vi "Dispersion measurements.vi"() -> ()   [LabVIEW 2015]
uses:
  <vilib>/express/express arith-compare/Formula/XNode/ExpressFormulaBlockNode.xnode
  <instrlib>/Rohde&Schwarz Vector Network Analyzer/Rohde&Schwarz Vector Network Analyzer.lvlib
panel:
  in  "Minimum field (Oe)":dbl min=-1000.0 max=1000.0
  in  "Maximum field (Oe)":dbl=1.0 min=0.0 max=1000.0
  out "Amplifier LinMag gain":dbl
  in  "Power amplifier LinMag gain (if 0, it will be calculated)":dbl min=0.0 max=20.0
  in  "Stop frequency (Hz)":dbl=15000000000.0 min=0.0 max=20000000000.0
  in  "Start frequency (Hz)":dbl=100000.0 min=0.0 max=20000000000.0
  in  "1 Hz < IFBW < 1MHz (10 kHz default)":dbl=10000.0 min=1.0 max=10000000.0
  in  "-20 dB < Power < 20 dB (0 dB default)":dbl min=-20.0 max=20.0
  in  "Delay time along ther sample (ps)":dbl min=0.0 max=1000.0
  out "DMM reading":dbl=5.649249
  out "Current field point":i32=98
  in  "DMM's connection":refnum<visa-resource-name>="Multimeter"
  in  "Choose the folder where the field dependencies of S-parameters and Z will be saved":path=path "C:/Users/ZJUcomposite/Desktop/Tests"
  in  "HMF's connection":refnum<visa-resource-name>="Generator"
  in  "VNA's connection":refnum<visa-resource-name>="ZNB-VNA"
  in  "Coil resistance > 0 (Ohm)":dbl=8.38 min=0.1 max=1000.0
  in  "Coil inductance > 0 (H)":dbl=0.32 min=0.0 max=100.0
  in  "Number of field points":i32=2 min=2 max=1000 step=1
  in  "Volltage to field coefficient > 0 (Oe/V)":dbl=4.29 min=0.0 max=1000.0
  in  "Max input voltage for the amplifier (0<V<2)":dbl=1.5 min=0.0 max=10.0
  in  "Number of frequency points":i32=5000 min=3 max=20000
  in  "VNA's port(s) used for measurements":string(combo)="S21"
  # "The procedure measures the frequency dispersions of S-parameters and Z for the specified magnetic fields.\n\nVNA must be already calibrated before the measurements. The procedure will not change the calibration but you can   modify IFBW and power. The frequency measurement range must be within the calibration range. \n\nThe measured fields must be within the maximum (+/-) field range.\n\nThe voltage to field coefficient (Oe/V) must be found from the coil calibration.\n\nThe delay time along the sample must be found separately.\n\nThe coil resistance R and inductance L must be larger than zero. Measure them by a digital multimeter (DMM).\n\nPlease check the maximum input voltage max V allowed for your waveform amplifier. Also the ratio maxV / R must be below the current rate of your waveform amplifier.  \n\n******************************************\nDmitriy Makhnovskiy@Hangzhou December 2018\nSensing Materials Technology Ltd, UK\nE-mail: contact@sensmattech.co.uk"
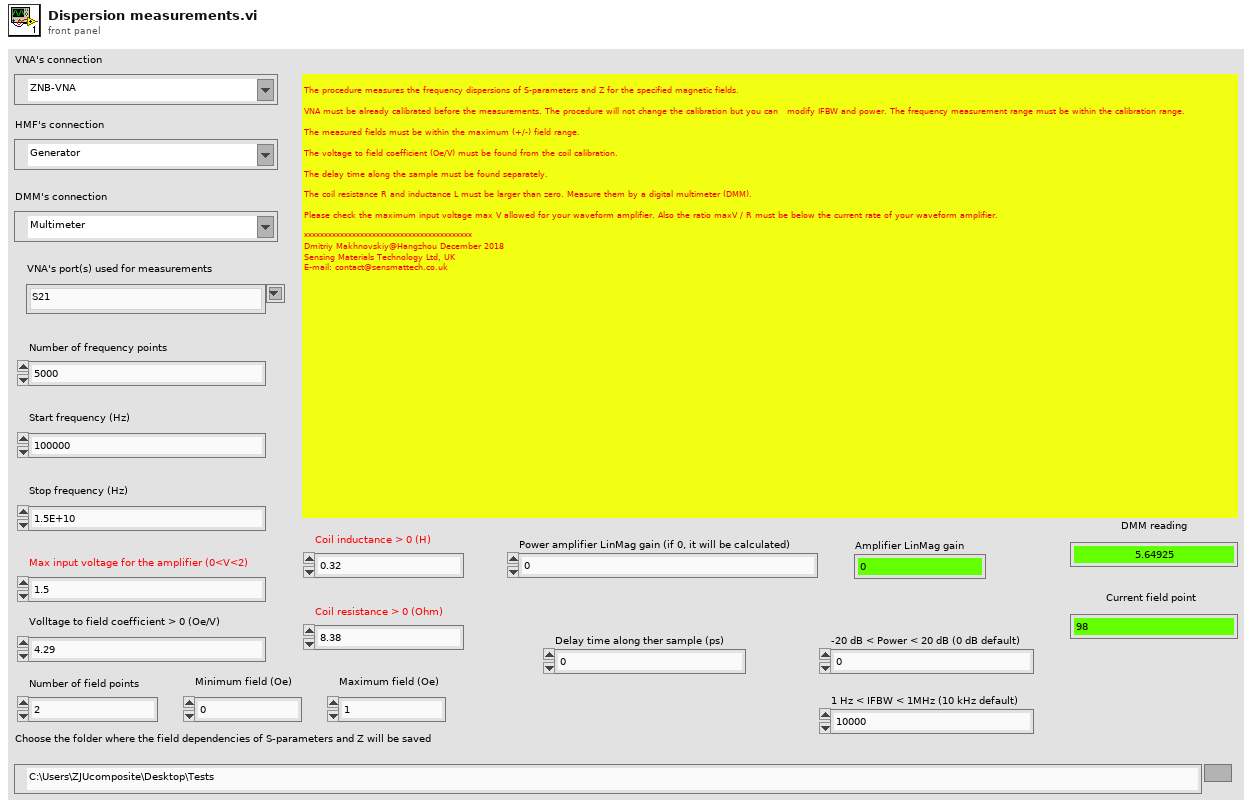
[diagram p1: front panel]
types:
  T1 = typedef "NI_Matrix.lvlib/RealMatrix.ctl" = dbl[][]
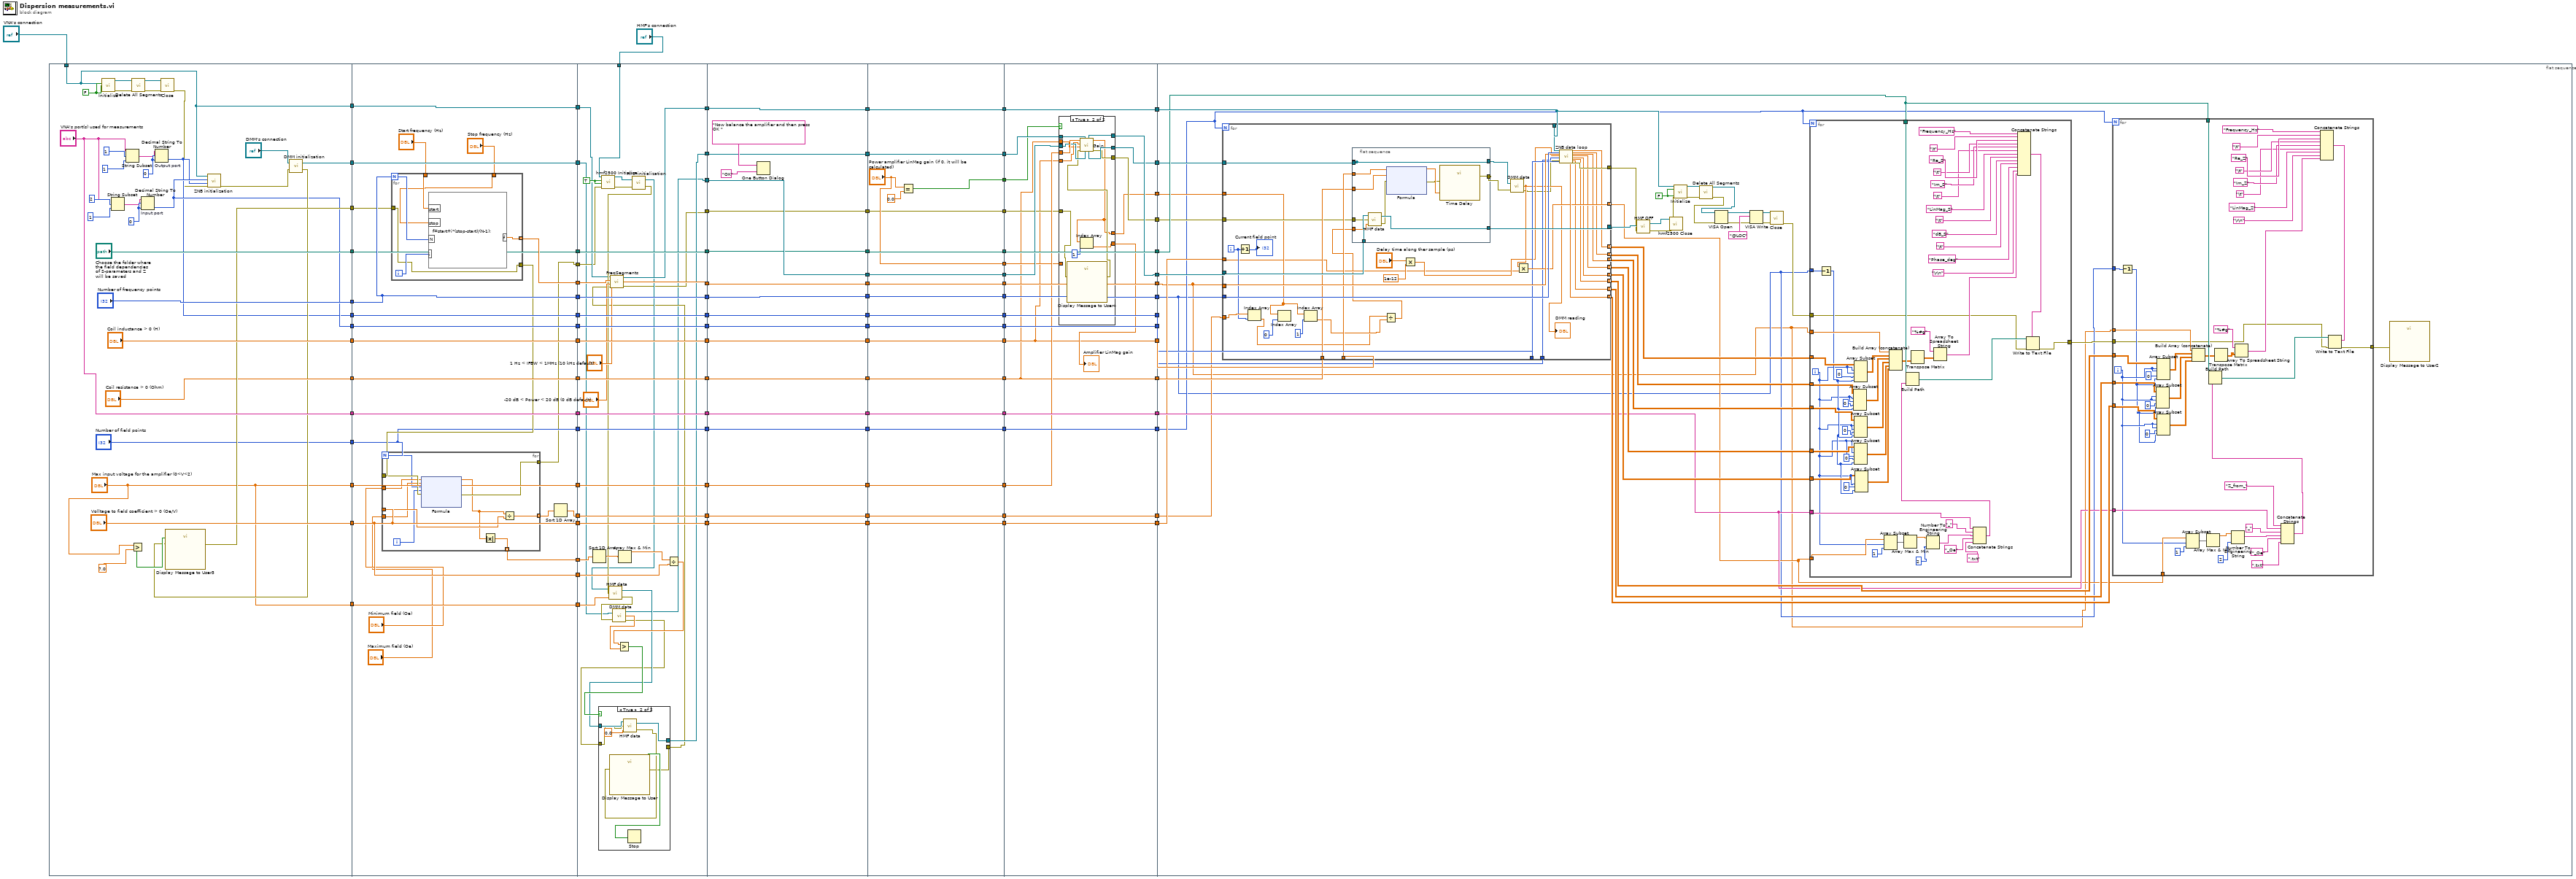
[diagram p0: block diagram]
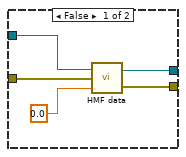
[diagram p2: hidden frame]
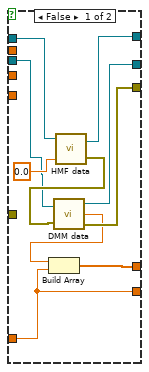
[diagram p3: hidden frame]
diagram:
  n1 = flat-sequence {
    tunnel: [w108] -> w92
    tunnel: ["VNA's port(s) used for measurements"] -> w89
    tunnel: "VNA's connection" -> [w108]
    tunnel: ["Number of frequency points"] -> w87
    tunnel: ["Coil inductance > 0 (H)"] -> w84
    tunnel: ["Coil resistance > 0 (Ohm)"] -> w81
    tunnel: ["Max input voltage for the amplifier (0<V<2)"] -> w78
    tunnel: ["Volltage to field coefficient > 0 (Oe/V)"] -> w75
    tunnel: ["Choose the folder where the field dependencies of S-parameters and Z will be saved"] -> w72
    tunnel: [w118] -> w71
    tunnel: [w113] -> w68
    tunnel: [w111] -> w65
    tunnel: [w110] -> w62
    tunnel: ["Number of field points"] -> w61
    tunnel: ["Max input voltage for the amplifier (0<V<2)"] -> w53
    tunnel: [w156] -> w100
    tunnel: [w153] -> w98
    tunnel: [w135] -> w96
    tunnel: [w155] -> w93
    tunnel: w92 -> [w155]
    tunnel: [w154] -> w90
    tunnel: w89 -> [w154]
    tunnel: w87 -> [w153]
    tunnel: [w152] -> w85
    tunnel: w84 -> [w152]
    tunnel: [w151] -> w82
    tunnel: w81 -> [w151]
    tunnel: [w139] -> w79
    tunnel: w78 -> [w139]
    tunnel: [w137] -> w76
    tunnel: w75 -> [w137]
    tunnel: [w150] -> w73
    tunnel: w72 -> [w150]
    tunnel: w71 -> [w146]
    tunnel: [w149] -> w69
    tunnel: w68 -> [w149]
    tunnel: [w148] -> w66
    tunnel: w65 -> [w148]
    tunnel: [w147] -> w63
    tunnel: w62 -> [w147]
    tunnel: w61 -> [w142]
    tunnel: [w142] -> w59
    tunnel: [w140] -> w57
    tunnel: [w138] -> w56
    tunnel: [w137] -> w55
    tunnel: [w136] -> w54
    tunnel: w53 -> [w136]
    tunnel: w100 -> [w214]
    tunnel: [w213] -> w99
    tunnel: w98 -> [w226]
    tunnel: [w226] -> w97
    tunnel: w96 -> [w194]
    tunnel: [w188] -> w95
    tunnel: [w212] -> w94
    tunnel: w93 -> [w196]
    tunnel: [w222] -> w91
    tunnel: w90 -> [w222]
    tunnel: "HMF's connection" -> [w195]
    tunnel: [w221] -> w86
    tunnel: w85 -> [w221]
    tunnel: [w220] -> w83
    tunnel: w82 -> [w220]
    tunnel: [w219] -> w80
    tunnel: w79 -> [w219]
    tunnel: [w218] -> w77
    tunnel: w76 -> [w218]
    tunnel: [w217] -> w74
    tunnel: w73 -> [w217]
    tunnel: [w198] -> w70
    tunnel: w69 -> [w190]
    tunnel: [w216] -> w67
    tunnel: w66 -> [w216]
    tunnel: [w215] -> w64
    tunnel: w63 -> [w215]
    tunnel: [w209] -> w60
    tunnel: w59 -> [w209]
    tunnel: [w208] -> w58
    tunnel: w57 -> [w208]
    tunnel: w56 -> [w205]
    tunnel: w55 -> [w204]
    tunnel: w54 -> [w202]
    tunnel: [w192] -> w3
    tunnel: w99 -> [w254]
    tunnel: [w254] -> w36
    tunnel: w97 -> [w253]
    tunnel: [w253] -> w34
    tunnel: w95 -> [w252]
    tunnel: [w252] -> w32
    tunnel: [w251] -> w30
    tunnel: w94 -> [w251]
    tunnel: [w250] -> w28
    tunnel: w91 -> [w250]
    tunnel: [w249] -> w26
    tunnel: w86 -> [w249]
    tunnel: [w248] -> w24
    tunnel: w83 -> [w248]
    tunnel: [w247] -> w22
    tunnel: w80 -> [w247]
    tunnel: [w246] -> w20
    tunnel: w77 -> [w246]
    tunnel: [w245] -> w18
    tunnel: w74 -> [w245]
    tunnel: [w244] -> w16
    tunnel: w70 -> [w244]
    tunnel: [w243] -> w14
    tunnel: w67 -> [w243]
    tunnel: [w242] -> w12
    tunnel: w64 -> [w242]
    tunnel: [w241] -> w10
    tunnel: w60 -> [w241]
    tunnel: [w240] -> w8
    tunnel: w58 -> [w240]
    tunnel: w3 -> [w239]
    tunnel: [w239] -> w2
    tunnel: w36 -> [w275]
    tunnel: [w275] -> w35
    tunnel: w34 -> [w274]
    tunnel: [w274] -> w33
    tunnel: w32 -> [w273]
    tunnel: [w273] -> w31
    tunnel: w30 -> [w272]
    tunnel: [w272] -> w29
    tunnel: w28 -> [w271]
    tunnel: [w271] -> w27
    tunnel: w26 -> [w270]
    tunnel: [w270] -> w25
    tunnel: w24 -> [w269]
    tunnel: [w269] -> w23
    tunnel: w22 -> [w268]
    tunnel: [w268] -> w21
    tunnel: w20 -> [w267]
    tunnel: [w267] -> w19
    tunnel: w18 -> [w266]
    tunnel: [w266] -> w17
    tunnel: w16 -> [w265]
    tunnel: [w265] -> w15
    tunnel: w14 -> [w264]
    tunnel: [w264] -> w13
    tunnel: w12 -> [w263]
    tunnel: [w263] -> w11
    tunnel: w10 -> [w262]
    tunnel: [w262] -> w9
    tunnel: w8 -> [w261]
    tunnel: [w261] -> w7
    tunnel: [w259] -> w6
    tunnel: ["Power amplifier LinMag gain (if 0, it will be calculated)"] -> w5
    tunnel: w2 -> [w257]
    tunnel: [w257] -> w1
    tunnel: w35 -> [w298]
    tunnel: [w298] -> w52
    tunnel: w33 -> [w297]
    tunnel: [w297] -> w51
    tunnel: w31 -> [w287]
    tunnel: [w285] -> w50
    tunnel: w29 -> [w296]
    tunnel: [w296] -> w49
    tunnel: w27 -> [w295]
    tunnel: [w295] -> w48
    tunnel: w25 -> [w277]
    tunnel: [w277] -> w47
    tunnel: w23 -> [w276]
    tunnel: [w276] -> w46
    tunnel: w21 -> [w286]
    tunnel: w19 -> [w294]
    tunnel: [w294] -> w45
    tunnel: w17 -> [w293]
    tunnel: [w293] -> w44
    tunnel: w15 -> [w288]
    tunnel: [w280] -> w43
    tunnel: w13 -> [w292]
    tunnel: [w292] -> w42
    tunnel: w11 -> [w291]
    tunnel: [w291] -> w41
    tunnel: w9 -> [w290]
    tunnel: [w290] -> w40
    tunnel: w7 -> [w289]
    tunnel: [w289] -> w39
    tunnel: [w284] -> w38
    tunnel: [w283] -> w37
    tunnel: w6 -> [w281]
    tunnel: w5 -> [w279]
    tunnel: w1 -> [w278]
    tunnel: w52 -> [w322]
    tunnel: w51 -> [w323]
    tunnel: w50 -> [w364]
    tunnel: w49 -> [w355]
    tunnel: w48 -> [w342]
    tunnel: w47 -> [w340]
    tunnel: w46 -> [w339]
    tunnel: w45 -> [w338]
    tunnel: w44 -> [w337]
    tunnel: w43 -> [w336]
    tunnel: w42 -> [w334]
    tunnel: w41 -> [w333]
    tunnel: w40 -> [w324]
    tunnel: w39 -> [w328]
    tunnel: w38 -> [w327]
    tunnel: w37 -> [w326]
    frame #0 {
      w124 = FALSE
      w132 = 0
      w128 = 0
      n2 = call <instrlib>:"Initialize.vi"("VISA resource name"=w108, "ID Query (T: Check)"=w124, "Reset (T: Reset)"=w124) -> ("VISA resource name out"=w104:refnum<visa-resource-name>, "error out"=w106:errorcluster)  [unwired: 11 in]
      n3 = String Subset(string="VNA's port(s) used for measurements", offset (0)=2, length (rest)=1) -> (substring=w131:string)
      n4 = String Subset(string="VNA's port(s) used for measurements", offset (0)=1, length (rest)=1) -> (substring=w127:string)
      n5 = Greater?(x="Max input voltage for the amplifier (0<V<2)", y=7.0) -> (0:w116:bool)
      n6 = call <instrlib>:"Delete All Segments.vi"("error in (no error)"=w106, "VISA resource name"=w104) -> ("error out"=w105:errorcluster, "VISA resource name out"=w103:refnum<visa-resource-name>)  [unwired: 8 in]
      n7 = Decimal String To Number "Input port"(string=w131, offset=w132, default (0L)=w132) -> (number=w111:i32)  [unwired: 1 out]
      n8 = Decimal String To Number "Output port"(string=w127, offset=w128, default (0L)=w128) -> (number=w110:i32)  [unwired: 1 out]
      n9 = call <instrlib>:"Close.vi"("error in (no error)"=w105, "VISA resource name"=w103) -> ("error out"=w107:errorcluster)  [unwired: 9 in]
      n10 = call "ZNB initialization.vi"("error in (no error)"=w107, "Output port"=w110, "Input port"=w111, "VISA resource name"=w108) -> ("error out"=w109:errorcluster)  [unwired: 7 in]
      n11 = call "DMM initialization.vi"("error in (no error)"=w109, "VISA resource name"="DMM's connection") -> ("error out"=w112:errorcluster, "VISA resource name out"=w113:refnum<visa-resource-name>)
      n12 = call "Display Message to User3"("error in (no error)"=w112, "Enable"=w116) -> ("error out"=w118:errorcluster)  [unwired: 8 in, 1 out]
    }
    frame #1 {
      n13 = for {
        N: w153 -> [w185]
        tunnel: [w184] -> w156 mode=indexing
        tunnel: w146 -> [w181]
        tunnel: "Start frequency (Hz)" -> [w183]
        tunnel: "Stop frequency (Hz)" -> [w182]
        tunnel: [w181] -> w143
        i -> [w186]
        n14 = formula code="f=start+i*(stop-start)/(N-1);"("start"=w183, "stop"=w182, "N"=w185, "i"=w186) -> ("f"=w184:dbl)
      }
      n15 = for {
        N: w142 -> [w158]
        tunnel: w143 -> [w163]
        tunnel: w137 -> [w166]
        tunnel: [w165] -> w141 mode=indexing
        tunnel: [w164] -> w138 mode=indexing
        tunnel: [w162] -> w135
        tunnel: "Minimum field (Oe)" -> [w160]
        tunnel: "Maximum field (Oe)" -> [w159]
        i -> [w157]
        n16 = xnode "Formula"("Min"=w160, "Max"=w159, "N"=w158, "i"=w157, "error in (no error)"=w163) -> ("Result"=w161:dbl, "error out"=w162:errorcluster)
        n17 = Absolute Value(x=w161) -> (abs(x)=w164:dbl)
        n18 = Divide(x=w161, y=w166) -> (x/y=w165:ext)
      }
      n19 = Sort 1D Array(array=w141) -> (sorted array=w140:ext[])
    }
    frame #2 {
      w225 = TRUE
      n20 = Sort 1D Array(array=w205) -> (sorted array=w206:dbl[])
      n21 = call <instrlib>:"hmf2500 Initialize.vi"("error in (no error)"=w194, "Reset (Reset)"=w225, "ID Query (Check)"=w225, "VISA resource name"=w195) -> ("error out"=w223:errorcluster, "VISA resource name out"=w224:refnum<visa-resource-name>)  [unwired: 6 in]
      n22 = Array Max & Min(array=w206) -> (max value=w207:dbl)  [unwired: 3 out]
      n23 = call "HMF initialization.vi"("error in (no error)"=w223, "VISA resource name"=w224) -> ("error out"=w203:errorcluster, "VISA resource name out"=w197:refnum<visa-resource-name>)
      n24 = call "HMF data.vi"("DC offset"=w202, "error in (no error)"=w203, "VISA resource name"=w197) -> ("error out"=w191:errorcluster, "VISA resource name out"=w199:refnum<visa-resource-name>)
      n25 = call "DMM data.vi"("VISA resource name"=w190, "error in (no error)"=w191) -> ("VISA resource name out"=w188:refnum<visa-resource-name>, "Voltage"=w189:dbl, "error out"=w187:errorcluster)
      n26 = Divide(x=w207, y=w204) -> (x/y=w201:dbl)
      n27 = Greater?(x=w201, y=w189) -> (0:w200:bool)
      n28 = case shown="True" w200 {
        tunnel: w199 -> [w230 w238]
        tunnel: w187 -> [w227 w235]
        tunnel: [w229 w232] -> w198
        tunnel: [w228 w233] -> w193
        frame False {
          n29 = call "HMF data.vi"("DC offset"=0.0, "error in (no error)"=w227, "VISA resource name"=w230) -> ("error out"=w228:errorcluster, "VISA resource name out"=w229:refnum<visa-resource-name>)
        }
        frame True {
          n30 = call "HMF data.vi"("DC offset"=0.0, "error in (no error)"=w235, "VISA resource name"=w238) -> ("error out"=w234:errorcluster, "VISA resource name out"=w232:refnum<visa-resource-name>)
          n31 = call "Display Message to User"("error in (no error)"=w234) -> ("error out"=w233:errorcluster, "OK"=w236:bool)  [unwired: 9 in]
          n32 = Stop(stop? (T)=w236) -> ()
        }
      }
      n33 = call "FreqSegments.vi"("VISA resource name"=w196, "FrequenciesIn"=w214, "Power"="-20 dB < Power < 20 dB (0 dB default)", "error in (no error)"=w193, "IFBW"="1 Hz < IFBW < 1MHz (10 kHz default)") -> ("VISA resource name out"=w212:refnum<visa-resource-name>, "FrequenciesOut"=w213:dbl[], "error out"=w192:errorcluster)
    }
    frame #3 {
      n34 = One Button Dialog(message="Now balance the amplifier and then press OK ", button name ("OK")="OK") -> ()  [unwired: 1 out]
    }
    frame #4 {
      n35 = Equal?(x="Power amplifier LinMag gain (if 0, it will be calculated)", y=0.0) -> (x = y?=w259:bool)
    }
    frame #5 {
      n36 = case shown="True" w281 {
        tunnel: w288 -> [w307 w318]
        tunnel: w287 -> [w304 w316]
        tunnel: w286 -> [_ w319]
        tunnel: [w306 w317] -> w285
        tunnel: [w303 w315] -> w280
        tunnel: [w302 w314] -> w284
        tunnel: [w299 w312] -> w283
        tunnel: [w300 w311] -> w282
        tunnel: w279 -> [w300 _]
        tunnel: w278 -> [_ w320]
        tunnel: w277 -> [_ w310]
        tunnel: w276 -> [_ w309]
        frame False {
          n37 = call "HMF data.vi"("DC offset"=0.0, "VISA resource name"=w307) -> ("error out"=w305:errorcluster, "VISA resource name out"=w306:refnum<visa-resource-name>)  [unwired: 1 in]
          n38 = call "DMM data.vi"("VISA resource name"=w304, "error in (no error)"=w305) -> ("VISA resource name out"=w303:refnum<visa-resource-name>, "Voltage"=w301:dbl, "error out"=w302:errorcluster)
          n39 = Build Array(w301, w300) -> (w299:dbl[])
        }
        frame True {
          n40 = call "Display Message to User4"("error in (no error)"=w320) -> ("error out"=w313:errorcluster)  [unwired: 9 in, 1 out]
          n41 = call "Gain.vi"("DMM VISA in"=w316, "HMF VISA in"=w318, "error in (no error)"=w313, "R"=w309, "L"=w310, "Max v input"=w319) -> ("error out"=w314:errorcluster, "Polynomial coeff"=w312:dbl[], "DMM VISA out"=w315:refnum<visa-resource-name>, "HMF VISA out"=w317:refnum<visa-resource-name>)  [unwired: 2 in]
          n42 = Index Array(array=w312, index=1) -> (element=w311:dbl)
        }
      }
      "Amplifier LinMag gain" <- w282
    }
    frame #6 {
      w353 = FALSE
      n43 = for {
        N: w324 -> [_]
        tunnel: w338 -> [w466]
        tunnel: w323 -> [w492]
        tunnel: [w488] -> w325 mode=indexing
        tunnel: w364 -> [w495]
        tunnel: [w494] -> w363
        tunnel: w355 -> [w493]
        tunnel: w322 -> [w491]
        tunnel: [w489] -> w343 mode=indexing
        tunnel: [w490] -> w335
        tunnel: [w487] -> w344 mode=indexing
        tunnel: [w486] -> w345 mode=indexing
        tunnel: [w485] -> w347 mode=indexing
        tunnel: [w484] -> w348 mode=indexing
        tunnel: [w483] -> w349 mode=indexing
        tunnel: [w482] -> w350 mode=indexing
        tunnel: [w481] -> w351 mode=indexing
        tunnel: w340 -> [w480]
        tunnel: w339 -> [w479]
        tunnel: w336 -> [w460]
        tunnel: w334 -> [w478]
        tunnel: w333 -> [w477]
        tunnel: w328 -> [w472]
        tunnel: w327 -> [w470]
        tunnel: w326 -> [w468]
        i -> [w471]
        n44 = Increment(x=w471) -> (x+1=→"Current field point":i32)
        n45 = Index Array(array=w472, index=w471) -> (element=w458:ext)
        n46 = Index Array(array=w468, index=0) -> ()  [unwired: 1 out]
        n47 = Index Array(array=w468, index=1) -> (element=w461:dbl)
        n48 = flat-sequence {
          tunnel: [w506] -> w494
          tunnel: w495 -> [w503]
          tunnel: [w502] -> w464
          tunnel: w480 -> [w501]
          tunnel: w479 -> [w500]
          tunnel: w470 -> [w498]
          tunnel: w465 -> [w497]
          tunnel: [w496] -> _
          tunnel: w460 -> [w496]
          tunnel: [w496] -> w459
          frame #0 {
            n49 = call "HMF data.vi"("DC offset"=w497, "error in (no error)"=w498, "VISA resource name"=w503) -> ("error out"=w499:errorcluster, "VISA resource name out"=w506:refnum<visa-resource-name>)
            n50 = xnode "Formula"("X1"=w501, "X2"=w500, "error in (no error)"=w499) -> ("Result"=w505:dbl, "error out"=w504:errorcluster)
            n51 = call "Time Delay"("error in (no error)"=w504, "Delay Time (s)"=w505) -> ("error out"=w502:errorcluster)  [unwired: 9 in]
          }
        }
        n52 = Divide(x=w458, y=w461) -> (x/y=w465:ext)
        n53 = Multiply(x="Delay time along ther sample (ps)", y=1e-12) -> (x*y=w474:dbl)
        n54 = call "DMM data.vi"("VISA resource name"=w459, "error in (no error)"=w464) -> ("Voltage"=w463:dbl, "error out"=w462:errorcluster)  [unwired: 1 out]
        "DMM reading" <- w463
        n55 = Multiply(x=w463, y=w466) -> (x*y=w488:ext)
        n56 = call "ZNB data loop.vi"("VISA resource name"=w493, "Number of frequency points"=w492, "Frequencies"=w491, "Delay Time"=w474, "Output Port"=w477, "Input Port"=w478, "error in (no error)"=w462) -> ("error out"=w490:errorcluster, "ReS"=w481:dbl[], "ImS"=w482:dbl[], "LinMagS"=w483:dbl[], "dBS"=w484:dbl[], "Phase"=w485:dbl[], "ReZ"=w486:dbl[], "ImZ"=w487:dbl[], "LinMagZ"=w489:dbl[])  [unwired: 12 in]
      }
      n57 = call "HMF OFF.vi"("error in (no error)"=w335, "VISA resource name"=w363) -> ("error out"=w361:errorcluster, "VISA resource name out"=w362:refnum<visa-resource-name>)
      n58 = call <instrlib>:"hmf2500 Close.vi"("error in (no error)"=w361, "VISA resource name"=w362) -> ("error out"=w354:errorcluster)  [unwired: 9 in]
      n59 = call <instrlib>:"Initialize.vi"("VISA resource name"=w355, "ID Query (T: Check)"=w353, "Reset (T: Reset)"=w353, "error in (no error)"=w354) -> ("VISA resource name out"=w331:refnum<visa-resource-name>, "error out"=w332:errorcluster)  [unwired: 10 in]
      n60 = call <instrlib>:"Delete All Segments.vi"("error in (no error)"=w332, "VISA resource name"=w331) -> ("error out"=w330:errorcluster, "VISA resource name out"=w329:refnum<visa-resource-name>)  [unwired: 8 in]
      n61 = VISA Open(error in (no error)=w330, VISA resource name=w329) -> (VISA resource name=w357:refnum<visa-resource-name>, error out=w356:errorcluster)  [unwired: 3 in]
      n62 = VISA Write(VISA resource name=w357, write buffer="@LOC", error in (no error)=w356) -> (VISA resource name out=w359:refnum<visa-resource-name>, error out=w358:errorcluster)  [unwired: 1 out]
      n63 = call <instrlib>:"Close.vi"("error in (no error)"=w358, "VISA resource name"=w359) -> ("error out"=w352:errorcluster)  [unwired: 9 in]
      n64 = for {
        N: w324 -> [_]
        tunnel: w352 -> [w410]
        tunnel: w325 -> [w456]
        tunnel: w351 -> [w457]
        tunnel: w322 -> [w453]
        tunnel: w323 -> [w449]
        tunnel: w342 -> [w422]
        tunnel: [w442] -> w346
        tunnel: w337 -> [w441]
        tunnel: w350 -> [w439]
        tunnel: w349 -> [w437]
        tunnel: w348 -> [w435]
        tunnel: w347 -> [w433]
        i -> [w414]
        n65 = Decrement(x=w449) -> (x-1=w415:i32)
        n66 = Array Subset(array=w439, index (row)=w414, length (row)=w414, index (col)=0, length (col)=w415) -> (w440:dbl[][])
        n67 = Array Subset(array=w457, index (row)=w414, length (row)=w414, index (col)=0, length (col)=w415) -> (w408:dbl[][])
        n68 = Array Subset(array=w437, index (row)=w414, length (row)=w414, index (col)=0, length (col)=w415) -> (w438:dbl[][])
        n69 = Array Subset(array=w435, index (row)=w414, length (row)=w414, index (col)=0, length (col)=w415) -> (w436:dbl[][])
        n70 = Array Subset(array=w433, index (row)=w414, length (row)=w414, index (col)=0, length (col)=w415) -> (w434:dbl[][])
        n71 = Array Subset(array=w456, index=w414, length=1) -> (w454:ext[])
        n72 = Build Array (concatenate)(w453, w408, w440, w438, w436, w434) -> (w409:T1)
        n73 = Array Max & Min(array=w454) -> (max value=w413:ext)  [unwired: 3 out]
        n74 = Transpose Matrix(1:w409) -> (0:w407:T1)
        n75 = Number To Engineering String(2:2, 4:w413) -> (0:w412:string)  [unwired: 2 in]
        n76 = Array To Spreadsheet String(array=w407, 3:"%#g") -> (spreadsheet string=w423:string)  [unwired: 1 in]
        n77 = Concatenate Strings(w422, "_", w412, "_Oe", ".txt") -> (w450:string)
        n78 = Build Path(base path=w441, name or relative path=w450) -> (appended path=w447:path)
        n79 = Concatenate Strings("Frequency_Hz", "\t", "Re_S", "\t", "Im_S", "\t", "LinMag_S", "\t", "dB_S", "\t", "Phase_deg", "\r\n", w423) -> (w446:string)
        n80 = Write to Text File(file (use dialog)=w447, text=w446, error in=w410) -> (error out=w442:errorcluster)  [unwired: 1 in, 2 out]
      }
      n81 = for {
        N: w324 -> [_]
        tunnel: w325 -> [w405]
        tunnel: w345 -> [w406]
        tunnel: w322 -> [w402]
        tunnel: w323 -> [w398]
        tunnel: w342 -> [w380]
        tunnel: [w391] -> w341
        tunnel: w337 -> [w390]
        tunnel: w344 -> [w388]
        tunnel: w343 -> [w386]
        tunnel: w346 -> [w367]
        i -> [w370]
        n82 = Decrement(x=w398) -> (x-1=w368:i32)
        n83 = Array Subset(array=w388, index (row)=w370, length (row)=w370, index (col)=0, length (col)=w368) -> (w389:dbl[][])
        n84 = Array Subset(array=w406, index (row)=w370, length (row)=w370, index (col)=0, length (col)=w368) -> (w401:dbl[][])
        n85 = Array Subset(array=w386, index (row)=w370, length (row)=w370, index (col)=0, length (col)=w368) -> (w387:dbl[][])
        n86 = Array Subset(array=w405, index=w370, length=1) -> (w403:ext[])
        n87 = Build Array (concatenate)(w402, w401, w389, w387) -> (w366:T1)
        n88 = Array Max & Min(array=w403) -> (max value=w375:ext)  [unwired: 3 out]
        n89 = Transpose Matrix(1:w366) -> (0:w365:T1)
        n90 = Number To Engineering String(2:2, 4:w375) -> (0:w374:string)  [unwired: 2 in]
        n91 = Array To Spreadsheet String(array=w365, 3:"%#g") -> (spreadsheet string=w377:string)  [unwired: 1 in]
        n92 = Concatenate Strings("Z_from_", w380, "_", w374, "_Oe", ".txt") -> (w399:string)
        n93 = Build Path(base path=w390, name or relative path=w399) -> (appended path=w396:path)
        n94 = Concatenate Strings("Frequency_Hz", "\t", "Re_Z", "\t", "Im_Z", "\t", "LinMag_Z", "\r\n", w377) -> (w395:string)
        n95 = Write to Text File(file (use dialog)=w396, text=w395, error in=w367) -> (error out=w391:errorcluster)  [unwired: 1 in, 2 out]
      }
      n96 = call "Display Message to User2"("error in (no error)"=w341) -> ()  [unwired: 9 in, 2 out]
    }
  }
